vi "Create TIFFs Folder.vi"(10 "Rev Path":path) -> (1 "Path To Exp":path, 2 "Path to TIFFS":path)   [LabVIEW 2020]
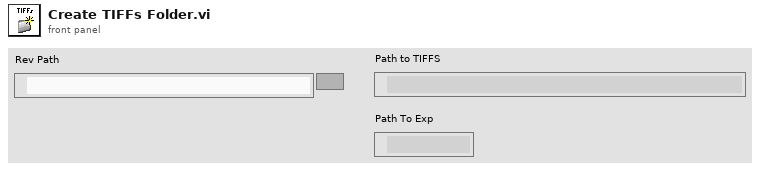
[diagram p1: front panel]
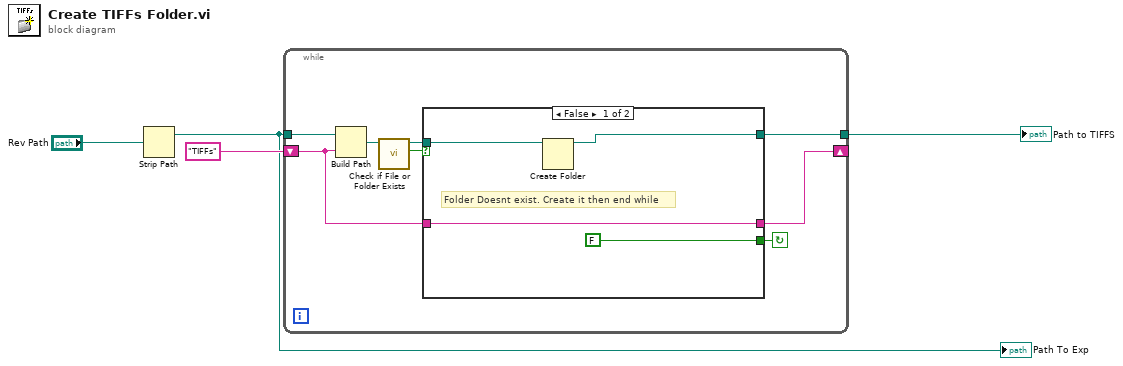
[diagram p0: block diagram]
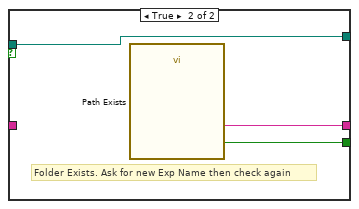
[diagram p2: hidden frame]
diagram:
  n1 = Strip Path(path="Rev Path") -> (stripped path=w1:path)  [unwired: 1 out]
  "Path To Exp" <- w1
  n2 = while {
    tunnel: [w8] -> w4
    shift-right: [w6] -> _
    shift-left: "TIFFs" ("name or relative path") -> [w5]
    tunnel: w1 -> [w7]
    stop <- w10 continue-if-true
    n3 = Build Path(base path=w7, name or relative path=w5) -> (appended path=w9:path)
    n4 = call <vilib>:"Check if File or Folder Exists.vi"("path"=w9) -> ("file or folder exists?"=w12:bool, "dup path"=w11:path)  [unwired: 8 in, 1 out]
    n5 = case shown="False" w12 {
      tunnel: w11 -> [w16 w17]
      tunnel: [FALSE ("Rename") w19] -> w10
      tunnel: [w15 w17] -> w8
      tunnel: [w14 w18] -> w6
      tunnel: w5 -> [w14 _]
      frame False {
        # "Folder Doesnt exist. Create it then end while"
        n6 = Create Folder(path (use dialog)=w16) -> (created path=w15:path)  [unwired: 2 in, 2 out]
      }
      frame True {
        # "Folder Exists. Ask for new Exp Name then check again"
        n7 = call "Path Exists"() -> ("NewName"=w18:string, "Rename"=w19:bool)  [unwired: 17 in, 1 out]
      }
    }
  }
  "Path to TIFFS" <- w4
